vi "StartStopApp.vi"(6 "Queues in":T1, 7 "PCtoMyRio in":T4, 8 "error in":errorcluster, 9 "On/Off":bool, 10 "References":T7, 11 "On/Off":refnum<vi>) -> (0 "error out":errorcluster, 2 "Queues out":T1, 3 "PCtoMyRio out":T4)   [LabVIEW 2019]
uses:
  Communication/TypeDef/#TypeDef_FromPCtoMR.ctl
  Communication/TypeDef/#TypeDef_Command.ctl
  Communication/TypeDef/#TypeDef_ErrorHandler_prop.ctl
  TypeDef/#TypeDef_References.ctl
  TypeDef/#TypeDef_Buttons.ctl
  TypeDef/#TypeDef_ReferencesMeassurementProp.ctl
  TypeDef/#TypeDef_ReferencesArchiveProp.ctl
  TypeDef/#TypeDef_Lists.ctl
  TypeDef/#TypeDef_MeasProp.ctl
  TypeDef/#TypeDef_OpProp.ctl
  TypeDef/#TypeDef_Enum_ModeOp.ctl
  Queue/TypeDef/#TypeDef_App_Queues.ctl
  TypeDef/#TypeDef_Enum_Buttons.ctl
  TypeDef/#TypeDef_EventStructureConstant.ctl
  TypeDef/#TypeDef_Enum_EventStructure.ctl
  Queue/TypeDef/#TypeDef_NetworkStream.ctl
  Communication/TypeDef/#TypeDef_FromMRtoPC.ctl
  Communication/TypeDef/#TypeDef_PropGraph.ctl
  Communication/TypeDef/#TypeDef_PropertiesToSave.ctl
  <vilib>/addons/database/Connection.llb/Conn ObjectReference.ctl
  Test/TypeDef/#TypeDef_DataToTest.ctl
  Communication/TypeDef/#TypeDef_SetGet.ctl
  Global_Freq.vi
  <vilib>/addons/database/NI_Database_API.lvlib
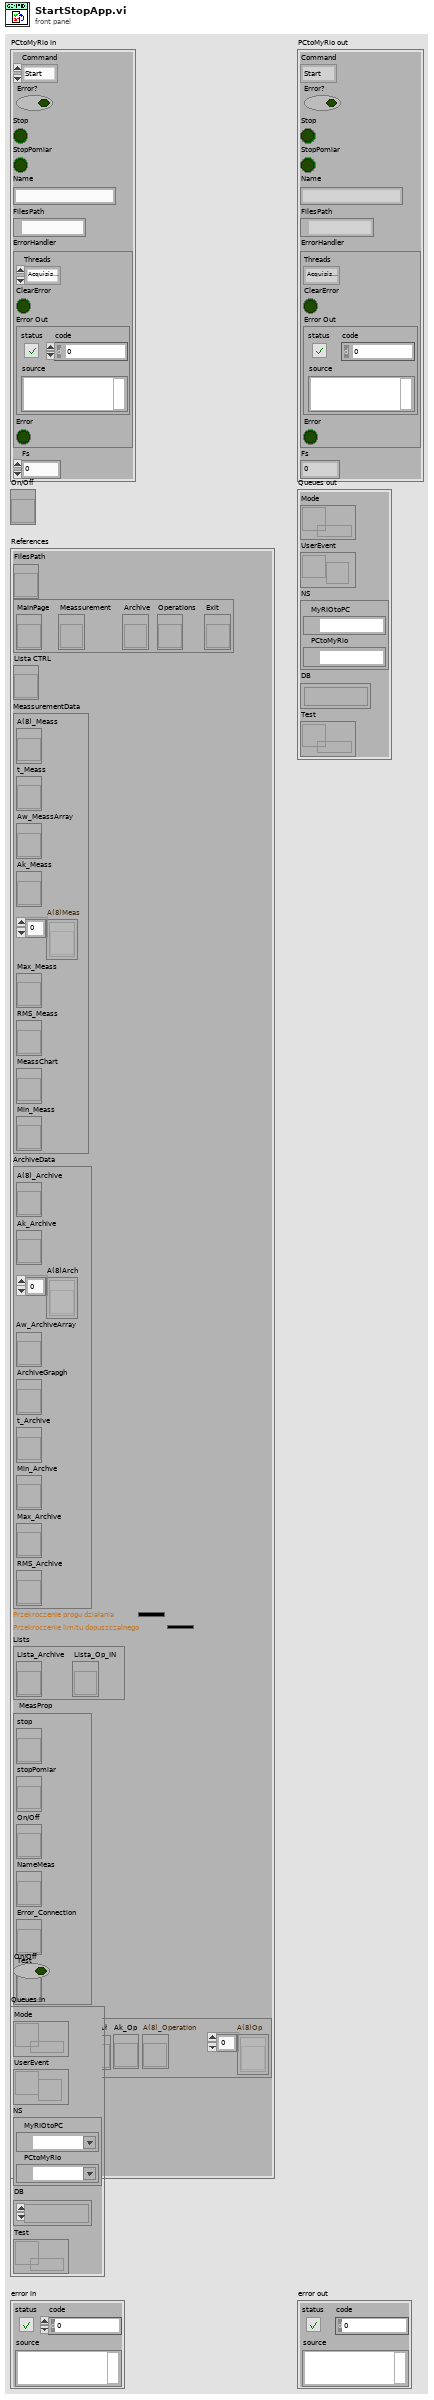
[diagram p1: front panel]
types:
  T1 = typedef "#TypeDef_App_Queues.ctl" = cluster{"Mode":refnum<queue>, "UserEvent":refnum<user-event>, "NS":T2, "DB":T3, "Test":refnum<queue>}
  T2 = typedef "#TypeDef_NetworkStream.ctl" = cluster{"MyRIOtoPC":refnum<k21>, "PCtoMyRio":refnum<k21>}
  T3 = typedef "NI_Database_API.lvlib/Conn ObjectReference.ctl" = refnum<k1>
  T4 = typedef "#TypeDef_FromPCtoMR.ctl" = cluster{"Command":T5, "Error?":bool, "Stop":bool, "StopPomiar":bool, "Name":string, "FilesPath":path, "ErrorHandler":T6, "Fs":dbl}
  T5 = typedef "#TypeDef_Command.ctl" = enum16{"Start", "End"}
  T6 = typedef "#TypeDef_ErrorHandler_prop.ctl" = cluster{"Threads":enum16{"Acquisistion", "Data Operation", "Save File"}, "ClearError":bool, "Error Out ":errorcluster, "Error":bool}
  T7 = typedef "#TypeDef_References.ctl" = cluster{"FilesPath":refnum<vi>, "MainButtons":T8, "Lista CTRL":refnum<vi>, "MeassurementData":T9, "ArchiveData":T10, "PD":u32, "LD":u32, "Lists":T11, "MeasProp":T12, "OpProp":T13, "DefaultColor":u32, "Tab Control":refnum<vi>}
  T8 = typedef "#TypeDef_Buttons.ctl" = cluster{"MainPage":refnum<vi>, "Meassurement":refnum<vi>, "Archive":refnum<vi>, "Operations":refnum<vi>, "Exit":refnum<vi>}
  T9 = typedef "#TypeDef_ReferencesMeassurementProp.ctl" = cluster{"A(8)_Meass":refnum<vi>, "t_Meass":refnum<vi>, "Aw_MeassArray":refnum<vi>, "Ak_Meass":refnum<vi>, "A(8)Meas":refnum<vi>[], "Max_Meass":refnum<vi>, "RMS_Meass":refnum<vi>, "MeassChart":refnum<vi>, "Min_Meass":refnum<vi>}
  T10 = typedef "#TypeDef_ReferencesArchiveProp.ctl" = cluster{"A(8)_Archive":refnum<vi>, "Ak_Archive":refnum<vi>, "A(8)Arch":refnum<vi>[], "Aw_ArchiveArray":refnum<vi>, "ArchiveGrapgh":refnum<vi>, "t_Archive":refnum<vi>, "Min_Archve":refnum<vi>, "Max_Archive":refnum<vi>, "RMS_Archive":refnum<vi>}
  T11 = typedef "#TypeDef_Lists.ctl" = cluster{"Lista_Archive":refnum<vi>, "Lista_Op_IN":refnum<vi>}
  T12 = typedef "#TypeDef_MeasProp.ctl" = cluster{"stop":refnum<vi>, "stopPomiar":refnum<vi>, "On/Off":refnum<vi>, "NameMeas":refnum<vi>, "Error_Connection":refnum<vi>, "Test":refnum<vi>}
  T13 = typedef "#TypeDef_OpProp.ctl" = cluster{"Name_Op":refnum<vi>, "t_Op":refnum<vi>, "Modu³":refnum<vi>, "Ak_Op":refnum<vi>, "A(8)_Operation":refnum<vi>, "A(8)Op":refnum<vi>[]}
  T14 = typedef "#TypeDef_DataToTest.ctl" = cluster{"FilesPath":path, "Name_Meas":string, "stop":bool, "Command":T5, "Fs":dbl, "Test":bool}
  T15 = typedef "#TypeDef_SetGet.ctl" = enum16{"Set", "Get"}
  T16 = typedef "#TypeDef_DBMode.ctl" = u16
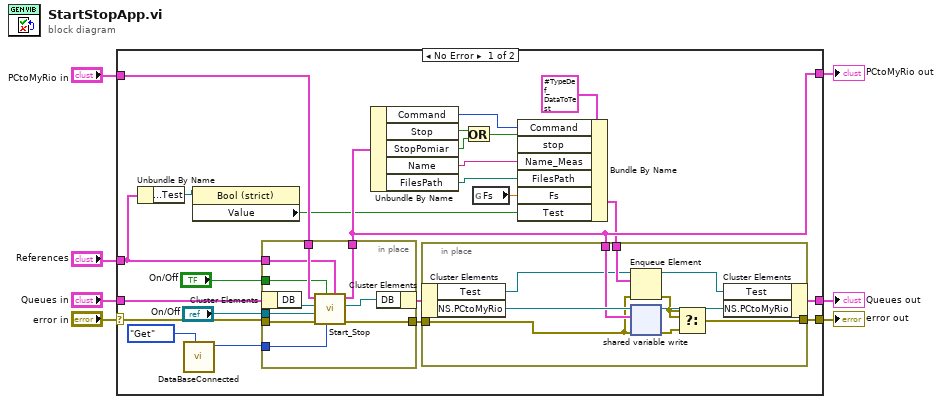
[diagram p0: block diagram]
diagram:
  n1 = case shown="No Error" "error in" {
    selector: "error in" -> [w22 w52]
    tunnel: [w19 w54] -> w7
    tunnel: "References" -> [w10 _]
    tunnel: "PCtoMyRio in" -> [w27 w54]
    tunnel: "Queues in" -> [w25 w53]
    tunnel: [w24 w52] -> w3
    tunnel: [w21 w53] -> w1
    frame No Error {
      n2 = Unbundle By Name(w10) -> ("MeasProp.Test"=w9:refnum<vi>)
      n3 = call "DataBaseConnected.vi"("Get/Set"=#TypeDef_SetGet."Get") -> ("BD out"=w31:T16)  [unwired: 10 in]
      n4 = property class="Bool (strict)"(reference=w9) -> ("Value"=w8:bool)  [unwired: 1 in, 2 out]
      n5 = in-place {
        in-place-border: w22 -> [w41]
        in-place-border: [w40] -> w29
        in-place-border: "On/Off" -> [w34]
        in-place-border: w27 -> [w37]
        in-place-border: [w36] -> w19
        in-place-border: "On/Off" -> [w35]
        in-place-border: w31 -> [w33]
        in-place-border: w10 -> [w32]
        n6 = in-place-cluster #1(w25) -> ("DB"=w39:T3)
        n7 = call "Start_Stop.vi"("References"=w32, "BD"=w33, "On/Off"=w35, "error in"=w41, "CtlRef"=w34, "DB in"=w39, "PCtoMyRio in"=w37) -> ("error out"=w40:errorcluster, "DB out"=w38:T3, "PCtoMyRio out"=w36:T4)  [unwired: 2 in]
        n8 = in-place-cluster #1("DB"=w38) -> (w26:T1)
      }
      n9 = Unbundle By Name(w19) -> ("Command"=w18:T5, "Stop"=w16:bool, "StopPomiar"=w17:bool, "Name"=w14:string, "FilesPath"=w13:path)
      n10 = Or(x=w16, y=w17) -> (x .or. y?=w15:bool)
      n11 = global read "Global_Freq.vi" "Fs"() -> (w12:dbl)
      n12 = Bundle By Name(cluster=T14 {"FilesPath"=path "", "Name_Meas"="", "stop"=FALSE, "Command"=enum."Start", "Fs"=1000.0, "Test"=FALSE}, "Command"=w18, "stop"=w15, "Name_Meas"=w14, "FilesPath"=w13, "Fs"=w12, "Test"=w8) -> (w11:T14)
      n13 = in-place {
        in-place-border: [w42] -> w24
        in-place-border: w19 -> [w50]
        in-place-border: w29 -> [w45]
        in-place-border: w11 -> [w49]
        n14 = in-place-cluster #2(w26) -> ("Test"=w47:refnum<queue>, "NS.PCtoMyRio"=w51:refnum<k21>)
        n15 = Enqueue Element(queue=w47, element=w49, error in (no error)=w45) -> (queue out=w48:refnum<queue>, error out=w44:errorcluster)  [unwired: 1 in, 1 out]
        n16 = shared-variable-write(w51, w45, w50) -> (w46:refnum<k21>, w43:errorcluster)  [unwired: 1 in, 1 out]
        n17 = Select(t=w44, s=w44, f=w43) -> (s? t:f=w42:errorcluster)
        n18 = in-place-cluster #2("Test"=w48, "NS.PCtoMyRio"=w46) -> (w21:T1)
      }
    }
    frame Error {
    }
  }
  "PCtoMyRio out" <- w7
  "error out" <- w3
  "Queues out" <- w1
